vi "Example-Supply.vi"() -> ()   [LabVIEW 2018]
panel:
  in  "停止":bool
  in  "Negative Output":bool=TRUE
  in  "Negative Voltage(V)":dbl=-3.0
  in  "Postivate Voltage(V)":dbl=3.0
  in  "Postivate Output":bool=TRUE
  out "returns":i32[](array[numeric])
  out "error out":errorcluster caption="错误输出"
  in  "error in (no error)":errorcluster caption="错误输入（无错误）"
  out "ftHandle out":u64=363562184
  in  "设备索引":i32
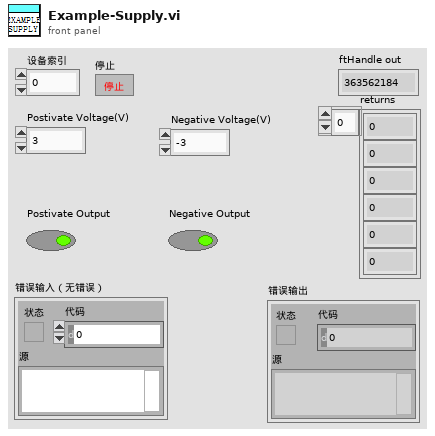
[diagram p1: front panel]
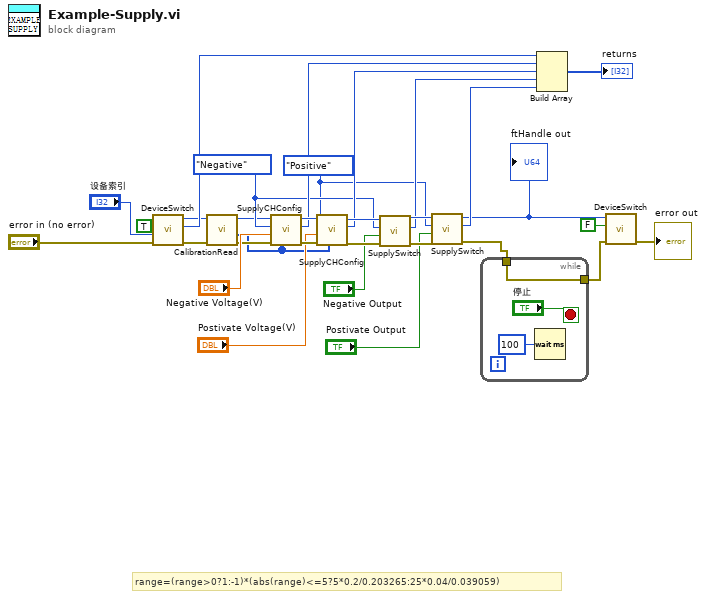
[diagram p0: block diagram]
diagram:
  w12 = enum16{"Positive", "Negative"}."Positive" ("CH")
  w13 = enum16{"Positive", "Negative"}."Negative" ("CH")
  # "range=(range>0?1:-1)*(abs(range)<=5?5*0.2/0.203265:25*0.04/0.039059)"
  n1 = call "DeviceSwitch.vi"("error in (no error)"="error in (no error)", "Device Index"="设备索引", "Open"=TRUE) -> ("error out"=w6:errorcluster, "function return"=w27:i32, "handle out"=w7:u64)  [unwired: 4 in, 2 out]
  n2 = call "CalibrationRead.vi"("handle"=w7, "error in (no error)"=w6) -> ("handle out"=w4:u64, "CalArray"=w3:u8[], "error out"=w5:errorcluster)  [unwired: 5 in, 1 out]
  n3 = call "SupplyCHConfig.vi"("CalArray"=w3, "error in (no error)"=w5, "Voltage(V)"="Negative Voltage(V)", "CH"=w13, "handle"=w4) -> ("error out"=w19:errorcluster, "function return"=w18:i32, "handle out"=w20:u64)  [unwired: 3 in, 1 out]
  n4 = call "SupplyCHConfig.vi"("CalArray"=w3, "error in (no error)"=w19, "Voltage(V)"="Postivate Voltage(V)", "CH"=w12, "handle"=w20) -> ("error out"=w24:errorcluster, "function return"=w17:i32, "handle out"=w21:u64)  [unwired: 3 in, 1 out]
  n5 = call "SupplySwitch.vi"("error in (no error)"=w24, "Output"="Negative Output", "CH"=w13, "handle"=w21) -> ("error out"=w23:errorcluster, "function return"=w16:i32, "handle out"=w22:u64)  [unwired: 5 in]
  n6 = call "SupplySwitch.vi"("error in (no error)"=w23, "Output"="Postivate Output", "CH"=w12, "handle"=w22) -> ("error out"=w2:errorcluster, "function return"=w15:i32, "handle out"=w14:u64)  [unwired: 5 in]
  "ftHandle out" <- w14
  n7 = while {
    tunnel: w2 -> [w34]
    tunnel: [w34] -> w1
    stop <- "停止" stop-if-true
    n8 = Wait (ms)(milliseconds to wait=u32 100 ("等待时间（毫秒）")) -> ()  [unwired: 1 out]
  }
  n9 = Build Array(w27, w18, w17, w16, w15) -> (→"returns":i32[])
  n10 = call "DeviceSwitch.vi"("error in (no error)"=w1, "Open"=FALSE, "handle"=w14) -> ("error out"=→"error out":errorcluster)  [unwired: 4 in, 4 out]
